vi "Config Synchronization Line.vi"(5 "Mode (Bypass)":T1(ring), 6 "Input Event":string="0", 7 "Line # (1)":u32=1 min=1 max=14, 8 "error in":errorcluster, 9 "Type (Digital I/O)":enum16{"Digital I/O", "TSP-Link"}(ring), 10 "Node In":string, 11 "VISA resource name":refnum<visa-resource-name>) -> (0 "error out":errorcluster, 2 "Node Out":string, 3 "VISA resource name out":refnum<visa-resource-name>, 4 "Command String":string)   [LabVIEW 2012, in "Keithley 2600 Series.lvlib"]
doc: "This VI will configure a synchronization line in the advanced trigger model.\n\n<b>Functions and Attributes Used</b>\ndigio.trigger[n].mode\ndigio.trigger[n].stimulus\ntsplink.trigger[n].mode\ntsplink.trigger[n].stimulus"
uses:
  Keithley 2600 Series.lvlib
  Private/GlobalVariables.vi
panel:
  # "(c) 2008 Keithley Instruments, Inc.  ALL RIGHTS RESERVED."
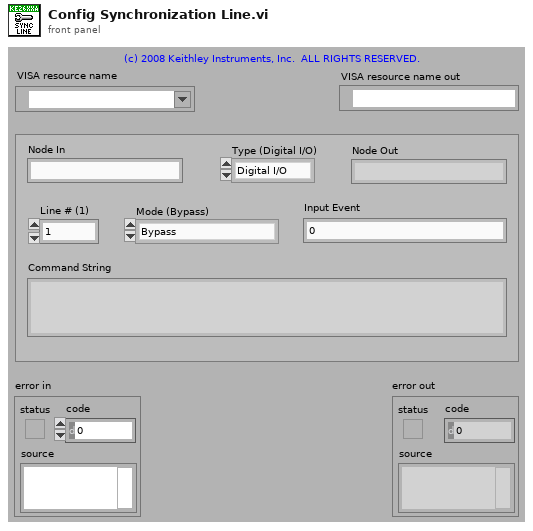
[diagram p1: front panel]
types:
  T1 = enum16{"Bypass", "Either", "Falling", "Rising", "Rising Acceptor", "Rising Master", "Synchronous", "Synchronous Acceptor", "Syncronous Master"}
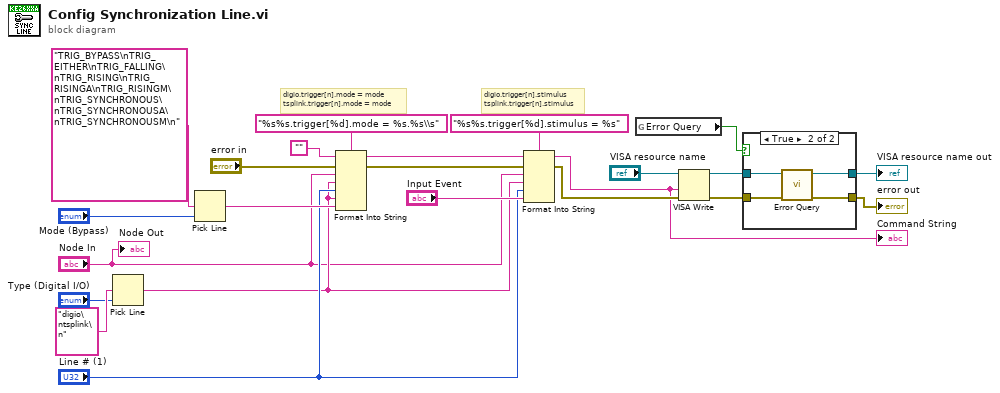
[diagram p0: block diagram]
diagram:
  # "digio.trigger[n].stimulus\ntsplink.trigger[n].stimulus"
  # "digio.trigger[n].mode = mode\ntsplink.trigger[n].mode = mode"
  n1 = Pick Line(multi-line string="digio\ntsplink\n", line index="Type (Digital I/O)") -> (output string=w13:string)  [unwired: 1 out]
  n2 = Pick Line(multi-line string="TRIG_BYPASS\nTRIG_EITHER\nTRIG_FALLING\nTRIG_RISING\nTRIG_RISINGA\nTRIG_RISINGM\nTRIG_SYNCHRONOUS\nTRIG_SYNCHRONOUSA\nTRIG_SYNCHRONOUSM\n", line index="Mode (Bypass)") -> (output string=w17:string)  [unwired: 1 out]
  n3 = Format Into String(format string="%s%s.trigger[%d].mode = %s.%s\\s", initial string="", error in="error in", "Node In", w13, "Line # (1)", w13, w17) -> (resulting string=w10:string, error out=w11:errorcluster)
  n4 = Format Into String(format string="%s%s.trigger[%d].stimulus = %s", initial string=w10, error in=w11, "Node In", w13, "Line # (1)", "Input Event") -> (resulting string=w2:string, error out=w8:errorcluster)
  "Command String" <- w2
  n5 = global read "GlobalVariables.vi" "Error Query"() -> (w1:bool)
  n6 = VISA Write(VISA resource name="VISA resource name", write buffer=w2, error in (no error)=w8) -> (VISA resource name out=w6:refnum<visa-resource-name>, error out=w5:errorcluster)  [unwired: 1 out]
  n7 = case shown="True" w1 {
    tunnel: w6 -> [w25 w29]
    tunnel: w5 -> [w24 w28]
    tunnel: [w25 w27] -> w4
    tunnel: [w24 w26] -> w3
    frame False {
    }
    frame True {
      n8 = call "Error Query.vi"("error in (no error)"=w28, "VISA resource name"=w29) -> ("error out"=w26:errorcluster, "VISA resource name out"=w27:refnum<visa-resource-name>)  [unwired: 8 out]
    }
  }
  "VISA resource name out" <- w4
  "error out" <- w3
  "Node Out" <- "Node In"
